vi "Initalization_DMM2831E.vi"(0 "error in (no error)":errorcluster) -> (1 "Instrument Out":refnum<visa-resource-name>, 2 "error out":errorcluster)   [LabVIEW 2023]
uses:
  <instrlib>/BK Precision 5491B/BK Precision 5491B.lvlib
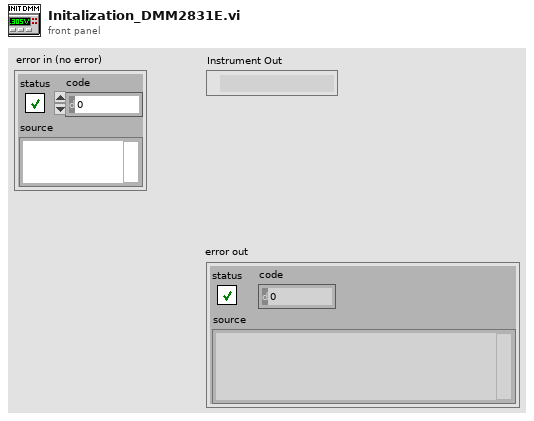
[diagram p1: front panel]
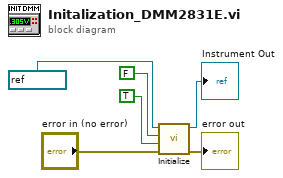
[diagram p0: block diagram]
diagram:
  n1 = call <instrlib>:"Initialize.vi"("error in (no error)"="error in (no error)", "Reset (True)"=TRUE, "ID Query (True)"=FALSE, "VISA resource name"=refnum<visa-resource-name> "DMM") -> ("error out"=→"error out":errorcluster, "VISA resource name out"=→"Instrument Out":refnum<visa-resource-name>)  [unwired: 6 in]
